vi "Verify Terminals for Message Type.vi"(7 "message type":T3, 8 "error in":errorcluster, 10 "directions":string[](array[string]), 11 "terminals":T1[](array[typedef])) -> (0 "error out":errorcluster, 2 "Tx terminal":T1, 3 "Rx terminal":T1)   [LabVIEW 2020, in "MIL-STD 1553 Import.lvlib"]
uses:
  MIL-STD 1553 Import.lvlib
  Shared/Message Type.ctl
  Shared/Terminal Endpoint.ctl
  Shared/Address.ctl
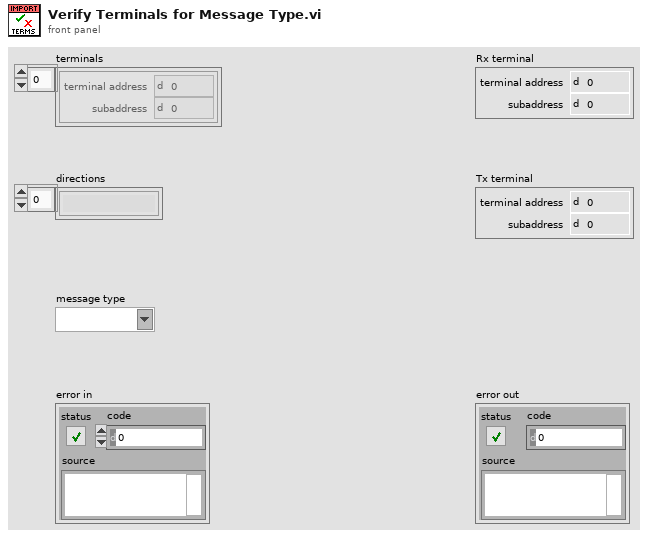
[diagram p1: front panel]
types:
  T1 = typedef "Terminal Endpoint.ctl" = cluster{"terminal address":T2, "subaddress":T2}
  T2 = typedef "Address.ctl" = u16
  T3 = typedef "Message Type.ctl" = string
  T4 = cluster{"terminal address":bool, "subaddress":bool}
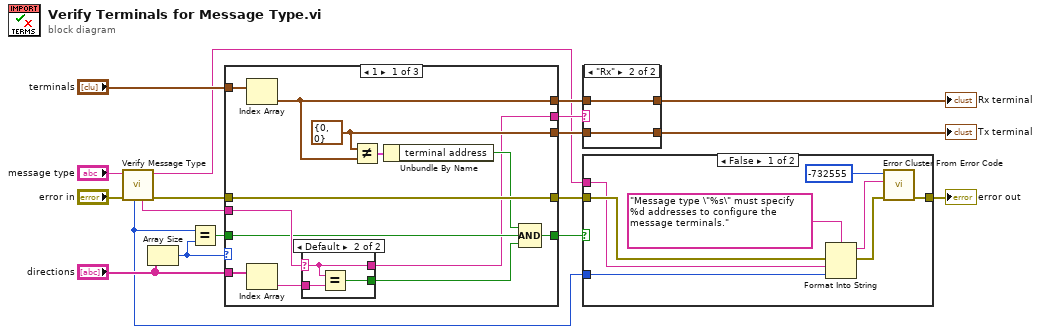
[diagram p0: block diagram]
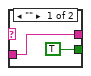
[diagram p4: hidden frame]
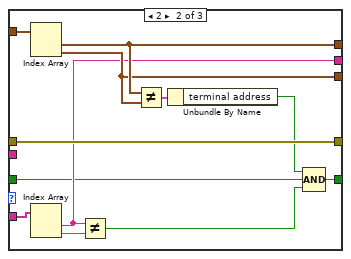
[diagram p5: hidden frame]
diagram:
  n1 = call "Verify Message Type.vi"("error in"="error in", "message type in"="message type") -> ("error out"=w8:errorcluster, "message type out"=w4:T3, "expected RT direction"=w10:string, "number of expected addresses"=w3:i32)  [unwired: 6 in]
  n2 = Array Size(array="directions") -> (size(s)=w7:i32)
  n3 = Equal?(x=w3, y=w7) -> (x = y?=w6:bool)
  n4 = case shown="1" w7 {
    tunnel: w8 -> [w27 w44 w49]
    tunnel: [w27 w44 w49] -> w1
    tunnel: "directions" -> [w31 w48 _]
    tunnel: "terminals" -> [w30 w47 _]
    tunnel: w10 -> [w26 _ _]
    tunnel: [w25 w43 _] -> w15
    tunnel: [w24 w42 _] -> w16
    tunnel: [w19 w41 _] -> w14
    tunnel: w6 -> [w22 w40 _]
    tunnel: [w20 w37 _] -> w5
    frame 1 {
      w24 = T1 {"terminal address"=0, "subaddress"=0} ("BC address")
      n5 = Index Array(array=w30) -> (element=w25:T1)  [unwired: 1 in]
      n6 = Index Array(array=w31) -> (element=w28:string)  [unwired: 1 in]
      n7 = case shown="Default" w26 {
        selector: w26 -> [_ w34]
        tunnel: w28 -> [w32 w36]
        tunnel: [TRUE w35] -> w21
        tunnel: [w32 w34] -> w19
        frame "" {
        }
        frame Default {
          n8 = Equal?(x=w34, y=w36) -> (x = y?=w35:bool)
        }
      }
      n9 = Not Equal?(x=w24, y=w25) -> (x != y?=w29:T4)
      n10 = Unbundle By Name(w29) -> ("terminal address"=w23:bool)
      n11 = Compound Arithmetic op=AND(w23, w22, w21) -> (w20:bool)
    }
    frame 2 {
      n12 = Index Array(array=w47) -> (element #1=w43:T1, element #2=w42:T1)  [unwired: 2 in]
      n13 = Index Array(array=w48) -> (element #1=w41:string, element #2=w45:string)  [unwired: 2 in]
      n14 = Not Equal?(x=w41, y=w45) -> (x != y?=w38:bool)
      n15 = Not Equal?(x=w43, y=w42) -> (x != y?=w46:T4)
      n16 = Unbundle By Name(w46) -> ("terminal address"=w39:bool)
      n17 = Compound Arithmetic op=AND(w39, w40, w38) -> (w37:bool)
    }
    frame Default {
    }
  }
  n18 = case shown="\"Rx\"" w14 {
    tunnel: w15 -> [w50 w53]
    tunnel: [w51 w53] -> w17
    tunnel: [w50 w52] -> w18
    tunnel: w16 -> [w51 w52]
    frame Default {
    }
    frame "Rx" {
    }
  }
  "Tx terminal" <- w18
  "Rx terminal" <- w17
  n19 = case shown="False" w5 {
    tunnel: w4 -> [w57 _]
    tunnel: w3 -> [w56 _]
    tunnel: [w54 w62] -> w2
    tunnel: w1 -> [w58 w62]
    frame False {
      n20 = Format Into String(format string="Message type \"%s\" must specify %d addresses to configure the message terminals.", error in=w58, w57, w56) -> (resulting string=w60:string, error out=w55:errorcluster)  [unwired: 1 in]
      n21 = call <vilib>:"Error Cluster From Error Code.vi"("error in (no error)"=w55, "error message (\"\")"=w60, "error code (0)"=-732555) -> ("error out"=w54:errorcluster)  [unwired: 6 in]
    }
    frame True {
    }
  }
  "error out" <- w2
